vi "mathoprators.vi"() -> ()   [LabVIEW 2019]
panel:
  out "divide":dbl
  out "mult":dbl
  out "sub":dbl
  out "add":dbl
  in  "Numeric 2":dbl
  in  "Numeric":dbl
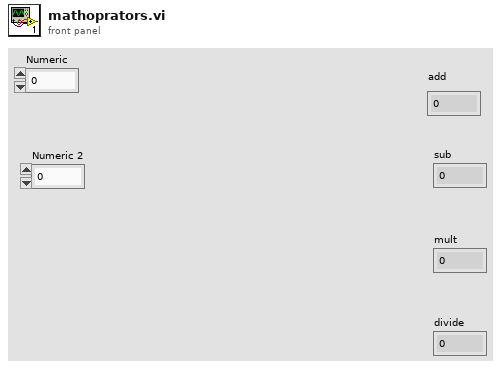
[diagram p1: front panel]
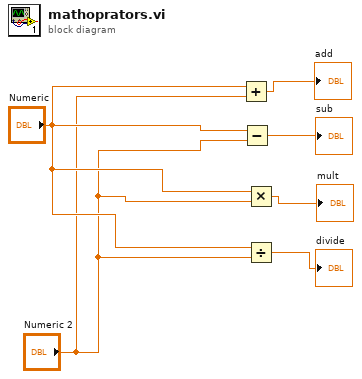
[diagram p0: block diagram]
diagram:
  n1 = Add(x="Numeric", y="Numeric 2") -> (x+y=→"add":dbl)
  n2 = Subtract(x="Numeric", y="Numeric 2") -> (x-y=→"sub":dbl)
  n3 = Multiply(x="Numeric", y="Numeric 2") -> (x*y=→"mult":dbl)
  n4 = Divide(x="Numeric", y="Numeric 2") -> (x/y=→"divide":dbl)
